vi "Close.vi"(0 "VI refnum in":refnum<vi>, 5 "Timeout before close":i32 caption="Timeout before close (0) [ms]" min=-1, 7 "Abort VI if necessary?":bool caption="Abort VI if necessary? (F)", 11 "Error in":errorcluster caption="Error in (no error)") -> (4 "VI path":path, 6 "Last execution state":T1(ring), 8 "VI aborted?":bool, 15 "Error out":errorcluster)   [LabVIEW 2017, in "VILauncher.lvlib"]
doc: "Closes the reference to the dynamic VI that <B>VI refnum in</B> refers to and returns the <B>VI path</B>.\n\nYou can set <B>Timeout before close</B> to something else than the default value of 0 to let this function wait for the dynamic VI to leave \"Run top level\" execution state before the VI refnum is closed. Set <B>Timeout before close</B> to -1 to wait indefinitely for the dynamic VI to stop executing. <B>Timeout before close</B> has a granularity of 20 ms.\n\nIf the optional <B>Abort VI if necessary?</B> is True (default is False), and the dynamic VI's execution state is \"Run top level\" even after <B>Timeout before close</B>, this function aborts the dynamic VI before the VI refnum is closed.\n\n<B>Last execution state</B> is the last value before the VI refnum was closed, but after an abort if such was executed.\n\nThe <B>VI aborted?</B> output will be True if the dynamic VI had to be aborted to get it out of \"Run top level\" execution state.\n\nThis VI is reentrant, and it runs even if there is an error on <B>Error in</B>. An error on <B>Error in</B> will not be overwritten by any error occurring in this function.\n\nSteen Schmidt\nGPower\n10/12 2013"
uses:
  VILauncher.lvlib
  Timing/GPTiming.lvlib
  Timing/Library/Wait/Wait_ms.vi
  Timing/Library/Remaining/Remaining_ms.vi
panel:
  # "Copyright © 2013\nGPower\nSee enclosed license file for terms and conditions"
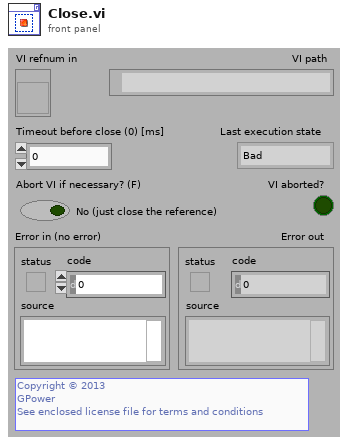
[diagram p1: front panel]
types:
  T1 = enum32{"Bad", "Idle", "Run top level", "Running"}
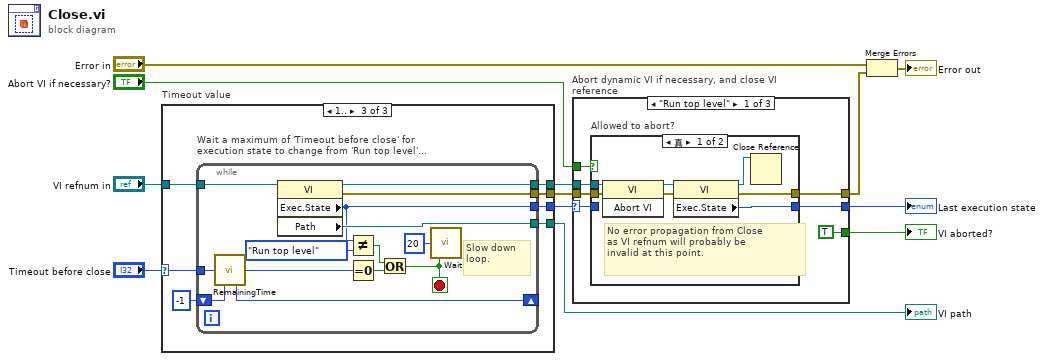
[diagram p0: block diagram]
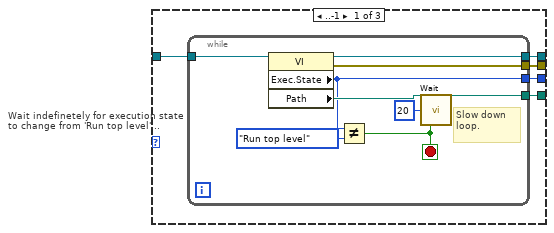
[diagram p2: hidden frame]
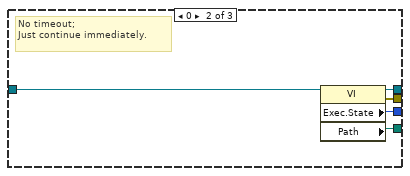
[diagram p3: hidden frame]
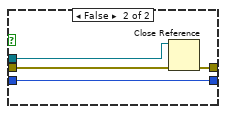
[diagram p4: hidden frame]
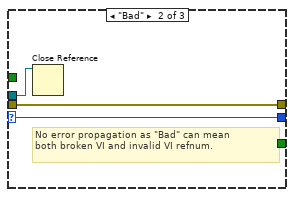
[diagram p5: hidden frame]
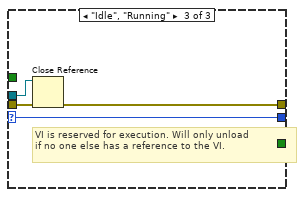
[diagram p6: hidden frame]
diagram:
  n1 = case "Timeout value" shown="1.." "Timeout before close" {
    selector: "Timeout before close" -> [_ _ w31]
    tunnel: "VI refnum in" -> [w17 w30 w37]
    tunnel: [w16 w29 w36] -> w7
    tunnel: [w15 w28 w35] -> w6
    tunnel: [w14 w27 w34] -> w5
    tunnel: [w13 w26 w33] -> w12
    frame ..-1 {
      n2 = while "Wait indefinetely for execution state\nto change from 'Run top level'..." {
        tunnel: w17 -> [w25]
        tunnel: [w24] -> w16
        tunnel: [w21] -> w15
        tunnel: [w23] -> w14
        tunnel: [w22] -> w13
        stop <- w18 stop-if-true
        # "Slow down\nloop."
        n3 = property class="VI"(reference=w25) -> (reference out=w24:refnum<vi>, error out=w23:errorcluster, "Exec.State"=w21:T1, "Path"=w22:path)  [unwired: 1 in]
        n4 = Not Equal?(x=w21, y=T1."Run top level") -> (x != y?=w18:bool)
        n5 = call-poly "Wait.vi"("Time to wait"=20 ("milliseconds to wait"), "Skip wait?"=w18) -> ()  [unwired: 13 in, 1 out]
      }
    }
    frame 0 {
      # "No timeout;\nJust continue immediately."
      n6 = property class="VI"(reference=w30) -> (reference out=w29:refnum<vi>, error out=w27:errorcluster, "Exec.State"=w28:T1, "Path"=w26:path)  [unwired: 1 in]
    }
    frame 1.. {
      n7 = while "Wait a maximum of 'Timeout before close' for\nexecution state to change from 'Run top level'..." {
        tunnel: w37 -> [w51]
        tunnel: [w50] -> w36
        tunnel: [w47] -> w35
        tunnel: [w49] -> w34
        tunnel: [w48] -> w33
        shift-right: [w40] -> _
        shift-left: i64 -1 ("Start time out") -> [w41]
        tunnel: w31 -> [w43]
        stop <- w39 stop-if-true
        # "Slow down\nloop."
        n8 = call-poly "RemainingTime.vi"("Time period target"=w43, "Start time in"=w41) -> ("Remaining time"=w42:i32, "Start time out"=w40:i64)  [unwired: 9 in, 3 out]
        n9 = property class="VI"(reference=w51) -> (reference out=w50:refnum<vi>, error out=w49:errorcluster, "Exec.State"=w47:T1, "Path"=w48:path)  [unwired: 1 in]
        n10 = Not Equal?(x=w47, y=T1."Run top level") -> (x != y?=w45:bool)
        n11 = Equal To 0?(x=w42) -> (x = 0?=w44:bool)
        n12 = Or(x=w45, y=w44) -> (x .or. y?=w39:bool)
        n13 = call-poly "Wait.vi"("Time to wait"=20 ("milliseconds to wait"), "Skip wait?"=w39) -> ()  [unwired: 13 in, 1 out]
      }
    }
  }
  "VI path" <- w12
  n14 = case "Abort dynamic VI if necessary, and close VI reference" shown="\"Run top level\"" w6 {
    selector: w6 -> [w52 w71 w73]
    tunnel: w7 -> [w58 w72 w75]
    tunnel: [w56 w70 w74] -> w1
    tunnel: w5 -> [w57 w70 w76]
    tunnel: [TRUE _ _] -> w10
    tunnel: [w55 w71 w73] -> w8
    tunnel: "Abort VI if necessary?" -> [w53 _ _]
    frame "Run top level" {
      n15 = case "Allowed to abort?" shown="真" w53 {
        tunnel: w58 -> [w65 w67]
        tunnel: w57 -> [w64 w68]
        tunnel: [w62 w66] -> w56
        tunnel: [w59 w69] -> w55
        tunnel: w52 -> [_ w69]
        frame True {
          # "No error propagation from Close\nas VI refnum will probably be\ninvalid at this point."
          n16 = invoke class="VI" method="Abort VI"(reference=w65, error in=w64) -> (reference out=w61:refnum<vi>, error out=w63:errorcluster)  [unwired: 1 in, 1 out]
          n17 = property class="VI"(reference=w61, error in=w63) -> (reference out=w60:refnum<vi>, error out=w62:errorcluster, "Exec.State"=w59:T1)
          n18 = Close Reference(reference=w60) -> ()  [unwired: 1 in, 1 out]
        }
        frame False {
          n19 = Close Reference(reference=w67, error in (no error)=w68) -> (error out=w66:errorcluster)
        }
      }
    }
    frame "Bad" {
      # "No error propagation as \"Bad\" can mean\nboth broken VI and invalid VI refnum."
      n20 = Close Reference(reference=w72) -> ()  [unwired: 1 in, 1 out]
    }
    frame "Idle", "Running" {
      # "VI is reserved for execution. Will only unload\nif no one else has a reference to the VI."
      n21 = Close Reference(reference=w75, error in (no error)=w76) -> (error out=w74:errorcluster)
    }
  }
  "Last execution state" <- w8
  "VI aborted?" <- w10
  n22 = Merge Errors("Error in", w1) -> (→"Error out":errorcluster)
